vi "Read DBL.vi"(8 "error in (no error)":errorcluster, 10 "# samples":i32, 11 "device handle in":T1) -> (0 "error out":errorcluster, 2 "Data":cdb[](array[numeric]), 3 "device handle out":T1)   [LabVIEW 2021, in "RTL-SDR.lvlib"]
uses:
  RTL-SDR.lvlib
  Controls/Device Handle.ctl
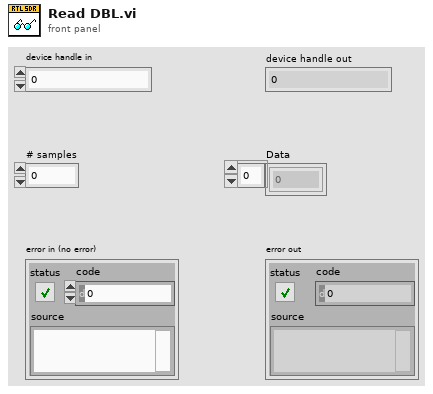
[diagram p1: front panel]
types:
  T1 = typedef "RTL-SDR.lvlib/Device Handle.ctl" = u64
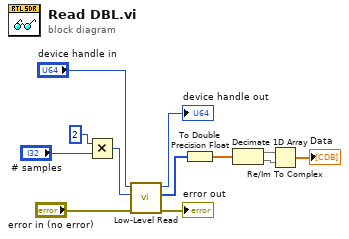
[diagram p0: block diagram]
diagram:
  n1 = Multiply(x=2, y="# samples") -> (x*y=w5:i32)
  n2 = call "Low-Level Read.vi"("error in (no error)"="error in (no error)", "# Samples to read"=w5, "device handle in"="device handle in") -> ("error out"=→"error out":errorcluster, "Samples"=w12:u8[], "device handle out"=→"device handle out":T1)  [unwired: 5 in, 1 out]
  n3 = To Double Precision Float(number=w12) -> (double precision float=w8:dbl[])
  n4 = Decimate 1D Array(w8) -> (w9:dbl[], w10:dbl[])
  n5 = Re/Im To Complex(1:w10, 2:w9) -> (0:→"Data":cdb[])
